vi "CorrectEyeResponse.vi"(8 "error in (no error)":errorcluster, 9 "y":dbl format="%0.2f", 10 "x":dbl format="%0.2f", 11 "TwoAfcEye in":refnum<class "TwoAfcEye.lvclass">) -> (0 "error out":errorcluster, 1 "Incorrect Response":bool, 2 "Correct Response":bool, 3 "TwoAfcEye out":refnum<class "TwoAfcEye.lvclass">)   [LabVIEW 2014, in "TwoAfcEye.lvclass"]
uses:
  TwoAfcEye.lvclass
  Trial Based Experiment Statechart/Trial Based Experiment.lvsc/State.ctl
  TwoAfcEye.lvclass/TwoAfcEye.ctl
  Trial Based Experiment Statechart/Trial Based Experiment.lvsc
panel:
  in  "State":T1
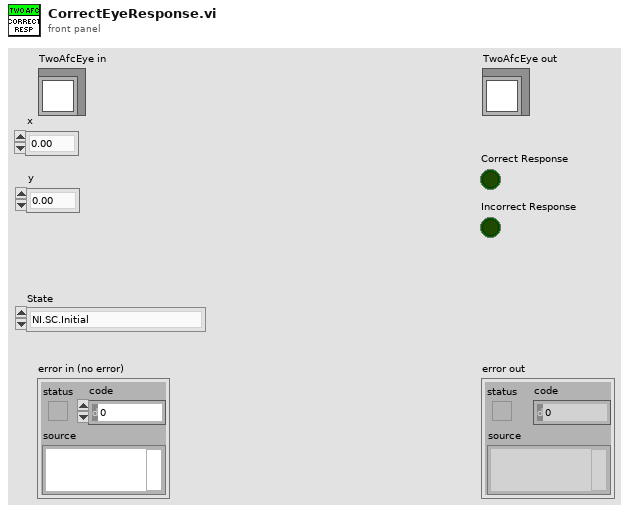
[diagram p1: front panel]
types:
  T1 = typedef "Trial Based Experiment.lvsc/State.ctl" = enum16{"NI.SC.Initial", "NI.SC.History", "NI.SC.ShallowHistory", "NI.SC.Terminal", "Cleanup", "State", "State\\Region\\Pause", "State\\Region\\Response Period", "State\\Region\\Delay Period", "State\\Region\\Hold Fixation", "State\\Region\\Acquire Fixation", "State\\Region\\Abort Trial", "State\\Region\\End Trial", "State\\Region\\Intertrial", "State\\Region\\Start Trial"}
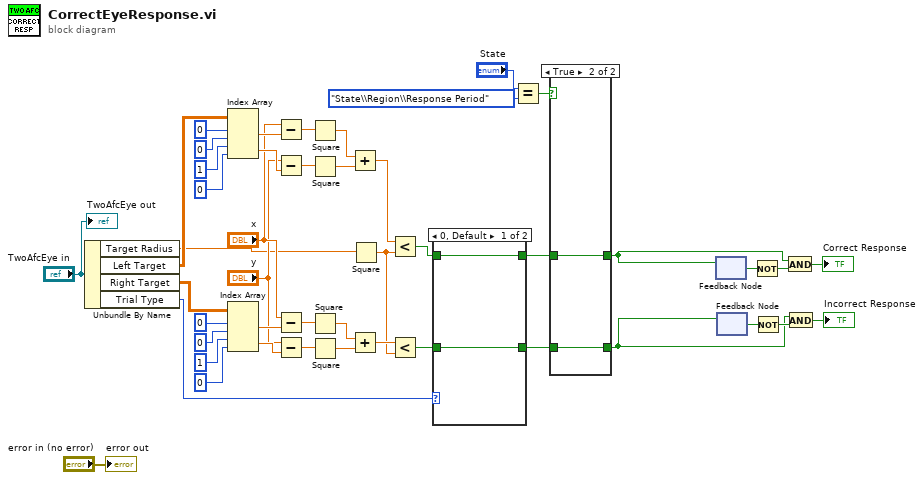
[diagram p0: block diagram]
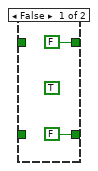
[diagram p2: hidden frame]
diagram:
  n1 = Unbundle By Name("TwoAfcEye in") -> ("Target Radius"=w14:dbl, "Left Target"=w16:dbl[][], "Right Target"=w15:dbl[][], "Trial Type"=w17:i32)
  n2 = Index Array(array=w16, index (row) #1=0 ("index"), index (col) #1=0 ("disabled index (col)"), index (row) #2=1 ("index"), index (col) #2=0 ("disabled index (col)")) -> (element #1=w26:dbl, element #2=w25:dbl)
  n3 = Index Array(array=w15, index (row) #1=0 ("index"), index (col) #1=0 ("disabled index (col)"), index (row) #2=1 ("index"), index (col) #2=0 ("disabled index (col)")) -> (element #1=w24:dbl, element #2=w23:dbl)
  n4 = Subtract(x="x", y=w26) -> (x-y=w37:dbl)
  n5 = Subtract(x="y", y=w25) -> (x-y=w36:dbl)
  n6 = Subtract(x="x", y=w24) -> (x-y=w35:dbl)
  n7 = Subtract(x="y", y=w23) -> (x-y=w38:dbl)
  n8 = Square(x=w37) -> (x^2=w33:dbl)
  n9 = Square(x=w36) -> (x^2=w34:dbl)
  n10 = Square(x=w35) -> (x^2=w31:dbl)
  n11 = Square(x=w38) -> (x^2=w32:dbl)
  n12 = Add(x=w33, y=w34) -> (x+y=w29:dbl)
  n13 = Add(x=w31, y=w32) -> (x+y=w30:dbl)
  n14 = Square(x=w14) -> (x^2=w22:dbl)
  n15 = Less?(x=w29, y=w22) -> (x < y?=w28:bool)
  n16 = Less?(x=w30, y=w22) -> (x < y?=w27:bool)
  n17 = case shown="0, Default" w17 {
    tunnel: [w48 w49] -> w21
    tunnel: w28 -> [w48 w50]
    tunnel: [w47 w50] -> w20
    tunnel: w27 -> [w47 w49]
    frame 0, Default {
    }
    frame 1 {
    }
  }
  n18 = Equal?(x="State", y=State."State\\Region\\Response Period" ("x")) -> (x = y?=w11:bool)
  n19 = case shown="True" w11 {
    tunnel: w21 -> [_ w54]
    tunnel: w20 -> [_ w53]
    tunnel: [FALSE w54] -> w6
    tunnel: [FALSE w53] -> w3
    frame False {
      (unwired) TRUE
    }
    frame True {
    }
  }
  n20 = feedback #1() -> (w5:bool)  [unwired: 1 in]
  n21 = feedback-in #1(w6) -> ()
  n22 = feedback #2() -> (w2:bool)  [unwired: 1 in]
  n23 = feedback-in #2(w3) -> ()
  n24 = Not(x=w5) -> (.not. x?=w8:bool)
  n25 = Not(x=w2) -> (.not. x?=w7:bool)
  n26 = And(x=w6, y=w8) -> (x .and. y?=→"Correct Response":bool)
  n27 = And(x=w3, y=w7) -> (x .and. y?=→"Incorrect Response":bool)
  "error out" <- "error in (no error)"
  "TwoAfcEye out" <- "TwoAfcEye in"
